vi "Demo1.vi"() -> ()   [LabVIEW 2014, in "SJ-210 Lib.lvlib"]
uses:
  SJ-210 Lib.lvlib
  Typedef/ACQ Data.ctl
  Typedef/Connection Data.ctl
panel:
  in  "Conection Data":T1={"VISA resource name"="COM4"}
  out "ACQ Data":T2
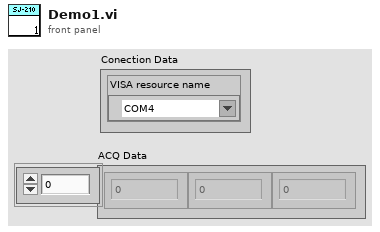
[diagram p1: front panel]
types:
  T1 = typedef "SJ-210 Lib.lvlib/Connection Data.ctl" = cluster{"VISA resource name":refnum<visa-resource-name>}
  T2 = typedef "SJ-210 Lib.lvlib/ACQ Data.ctl" = sgl[]
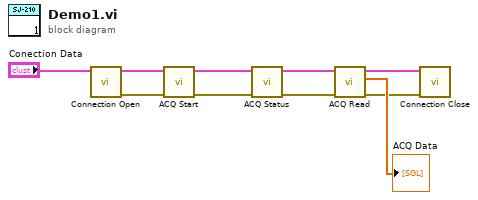
[diagram p0: block diagram]
diagram:
  n1 = call "Connection Open.vi"("Conection Data"="Conection Data") -> ("error out"=w7:errorcluster, "Conection Data Out"=w8:T1)  [unwired: 9 in]
  n2 = call "ACQ Start.vi"("error in (no error)"=w7, "Conection Data"=w8) -> ("error out"=w3:errorcluster, "Conection Data Out"=w4:T1)  [unwired: 8 in]
  n3 = call "ACQ Status.vi"("error in (no error)"=w3, "Conection Data"=w4) -> ("error out"=w2:errorcluster, "Conection Data Out"=w1:T1)  [unwired: 8 in]
  n4 = call "ACQ Read.vi"("error in (no error)"=w2, "Conection Data"=w1) -> ("error out"=w5:errorcluster, "ACQ Data"=→"ACQ Data":T2, "Conection Data Out"=w6:T1)  [unwired: 7 in]
  n5 = call "Connection Close.vi"("error in (no error)"=w5, "Conection Data"=w6) -> ()  [unwired: 8 in, 2 out]
